vi "FolderNameMatch.vi"(2 "Order":string[](array[string])=["baseline1_", "training1_", "training2_", "training3_", "training4_", "training5_", "training6_", "training7_", "training8_", "training9_", "training10_", "post1_", "post2_"], 3 "Input":string[](array[string])) -> (1 "Output":string[](array[string]))   [LabVIEW 2015]
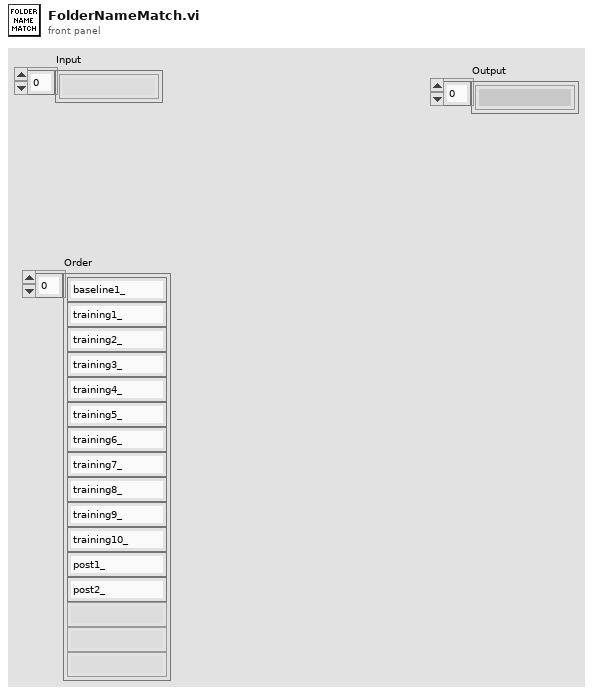
[diagram p1: front panel]
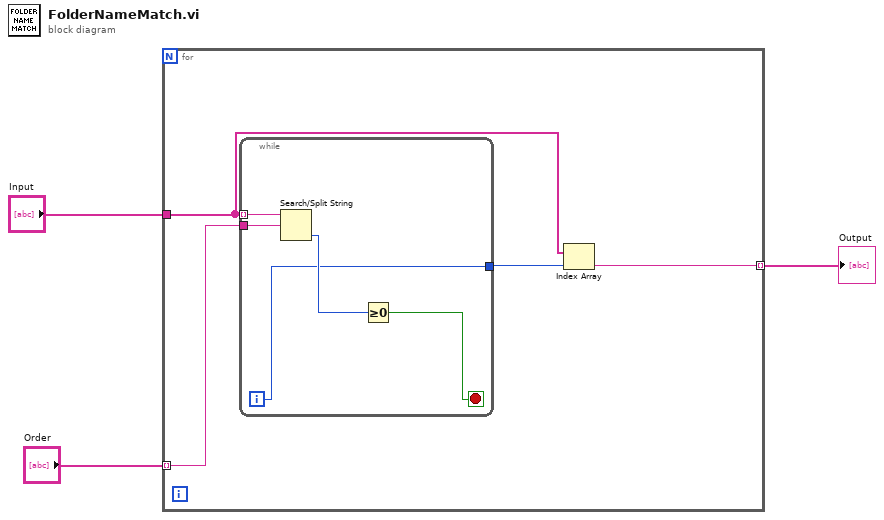
[diagram p0: block diagram]
diagram:
  n1 = for {
    tunnel: "Order" -> [w7] mode=indexing
    tunnel: "Input" -> [w6]
    tunnel: [w4] -> w1 mode=indexing
    n2 = while {
      tunnel: w6 -> [w12] mode=indexing
      tunnel: w7 -> [w11]
      tunnel: [w8] -> w5
      i -> [w8]
      stop <- w9 stop-if-true
      n3 = Search/Split String(string=w12, search string/char (-)=w11) -> (offset of match=w10:i32)  [unwired: 1 in, 2 out]
      n4 = Greater Or Equal To 0?(x=w10) -> (x >= 0?=w9:bool)
    }
    n5 = Index Array(array=w6, index=w5) -> (element=w4:string)
  }
  "Output" <- w1
